vi "LaserPIDPositioning.vi"(0 "Servo Device In":i32, 1 "Vertical Edge":T1 {"Point2 (Real-World)"."Y" format="%.2f"; "Point2 (Real-World)"."X" format="%.2f"; "Point1 (Real-World)"."Y" format="%.2f"; "Point1 (Real-World)"."X" format="%.2f"; "Point2 (Pixels)"."Y" format="%.2f"; "Point2 (Pixels)"."X" format="%.2f"; "Point1 (Pixels)"."Y" format="%.2f"; "Point1 (Pixels)"."X" format="%.2f"}, 2 "Horizontal Edge":T1 {"Point2 (Real-World)"."Y" format="%.2f"; "Point2 (Real-World)"."X" format="%.2f"; "Point1 (Real-World)"."Y" format="%.2f"; "Point1 (Real-World)"."X" format="%.2f"; "Point2 (Pixels)"."Y" format="%.2f"; "Point2 (Pixels)"."X" format="%.2f"; "Point1 (Pixels)"."Y" format="%.2f"; "Point1 (Pixels)"."X" format="%.2f"}, 4 "servo error in":errorcluster, 5 "error in":errorcluster, 8 "Destination Point":cluster{"DestinationX":dbl, "DestinationY":dbl}, 9 "Servo Angles In":cluster{"Angle X":dbl, "Angle Y":dbl}) -> (11 "Servo Angles Out":cluster{"Angle X":dbl, "Angle Y":dbl}, 14 "Servo Device Out":i32, 18 "servo error out":errorcluster, 19 "error out":errorcluster)   [LabVIEW 2014]
uses:
  <vilib>/addons/control/pid/pid.llb/PID (DBL).vi
  <vilib>/vision/NI_Vision_Development_Module.lvlib
  <vilib>/addons/control/pid/NI_PID_pid.lvlib
panel:
  out "x+y 2":dbl
  out "x+y":dbl
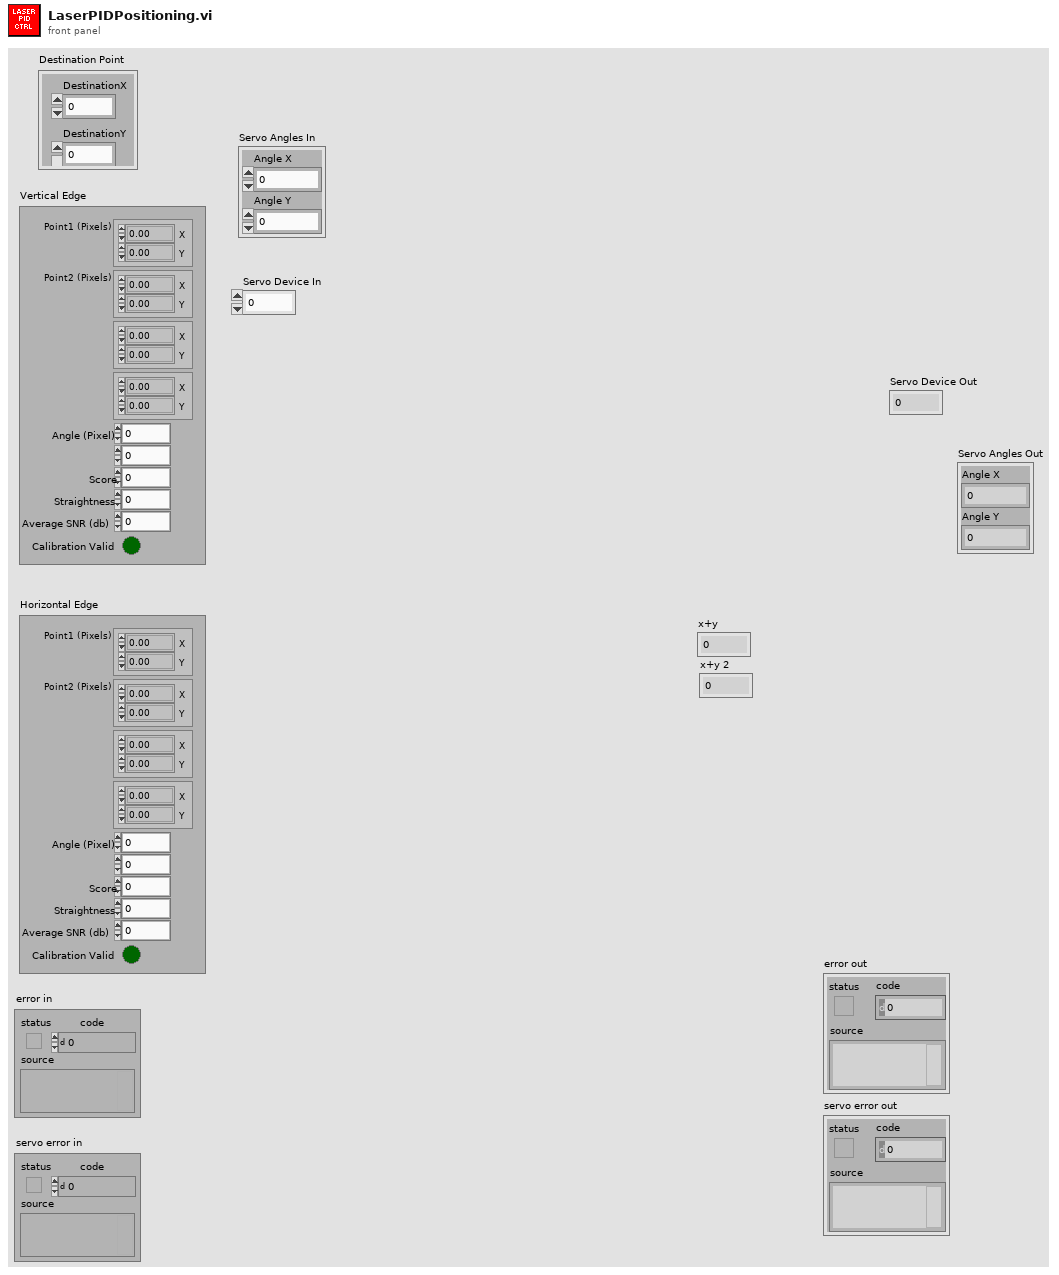
[diagram p1: front panel]
types:
  T1 = cluster{"Point1 (Pixels)":cluster{"X":sgl, "Y":sgl}, "Point2 (Pixels)":cluster{"X":sgl, "Y":sgl}, "Point1 (Real-World)":cluster{"X":sgl, "Y":sgl}, "Point2 (Real-World)":cluster{"X":sgl, "Y":sgl}, "Angle (Pixel)":dbl, "Angle (Real-World)":dbl, "Score":dbl, "Straightness":dbl, "Average SNR (db)":dbl, "Calibration Valid":bool}
  T2 = cluster{"proportional gain (Kc)":dbl, "integral time (Ti, min)":dbl, "derivative time (Td, min)":dbl}
  T3 = cluster{cluster{"X":sgl, "Y":sgl}, cluster{"X":sgl, "Y":sgl}}
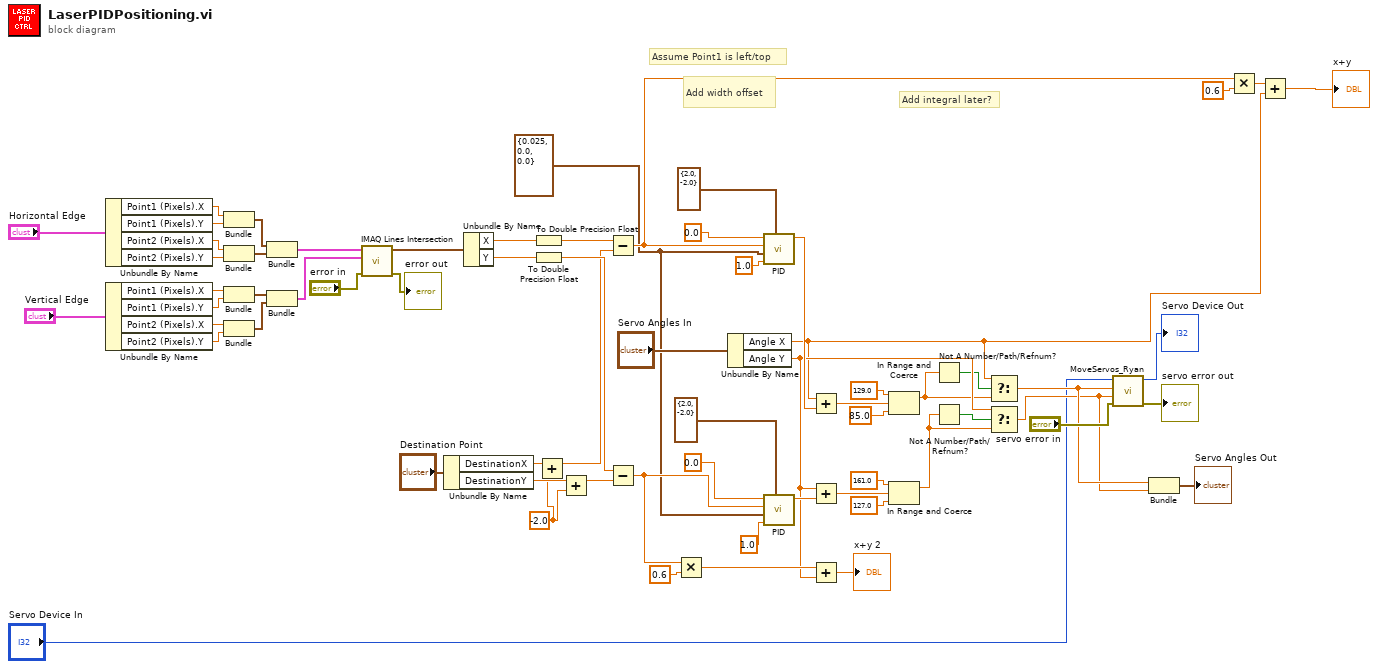
[diagram p0: block diagram]
diagram:
  w1 = -2.0 ("y")
  w4 = T2 {"proportional gain (Kc)"=0.025, "integral time (Ti, min)"=0.0, "derivative time (Td, min)"=0.0} ("PID gains")
  # "Add integral later?"
  # "Add width offset"
  # "Assume Point1 is left/top"
  n1 = Unbundle By Name("Horizontal Edge") -> ("Point1 (Pixels).X"=w63:sgl, "Point1 (Pixels).Y"=w62:sgl, "Point2 (Pixels).X"=w61:sgl, "Point2 (Pixels).Y"=w60:sgl)
  n2 = Unbundle By Name("Vertical Edge") -> ("Point1 (Pixels).X"=w54:sgl, "Point1 (Pixels).Y"=w53:sgl, "Point2 (Pixels).X"=w52:sgl, "Point2 (Pixels).Y"=w51:sgl)
  n3 = Bundle("X"=w63, "Y"=w62) -> (w59:cluster{"X":sgl, "Y":sgl})  [unwired: 1 in]
  n4 = Bundle("X"=w61, "Y"=w60) -> (w58:cluster{"X":sgl, "Y":sgl})  [unwired: 1 in]
  n5 = Bundle("X"=w54, "Y"=w53) -> (w56:cluster{"X":sgl, "Y":sgl})  [unwired: 1 in]
  n6 = Bundle("X"=w52, "Y"=w51) -> (w55:cluster{"X":sgl, "Y":sgl})  [unwired: 1 in]
  n7 = Bundle(w59, w58) -> (w57:T3)  [unwired: 1 in]
  n8 = Bundle(w56, w55) -> (w50:T3)  [unwired: 1 in]
  n9 = call "IMAQ Lines Intersection"("error in (no error)"="error in", "Line 2"=w50, "Line 1"=w57) -> ("error out"=→"error out":errorcluster, "Intersection Point"=w48:cluster{"X":sgl, "Y":sgl})  [unwired: 6 in, 1 out]
  n10 = Unbundle By Name("Destination Point") -> ("DestinationX"=w45:dbl, "DestinationY"=w41:dbl)
  n11 = Unbundle By Name(w48) -> ("X"=w38:sgl, "Y"=w42:sgl)
  n12 = To Double Precision Float(number=w38) -> (double precision float=w27:dbl)
  n13 = To Double Precision Float(number=w42) -> (double precision float=w37:dbl)
  n14 = Add(x=w45, y=w1) -> (x+y=w3:dbl)
  n15 = Add(x=w41, y=w1) -> (x+y=w2:dbl)
  n16 = Subtract(x=w27, y=w3) -> (x-y=w25:dbl)
  n17 = Subtract(x=w37, y=w2) -> (x-y=w22:dbl)
  n18 = Multiply(x=w22, y=0.6) -> (x*y=w21:dbl)
  n19 = Unbundle By Name("Servo Angles In") -> ("Angle X"=w10:dbl, "Angle Y"=w13:dbl)
  n20 = call-poly <vilib>:"PID.vi"("output range"=cluster{"output high":dbl, "output low":dbl} {"output high"=2.0, "output low"=-2.0}, "dt (s)"=1.0, "PID gains"=w4, "process variable"=w25, "setpoint"=0.0) -> ("output"=w16:dbl)  [unwired: 5 in, 1 out]
  n21 = call-poly <vilib>:"PID.vi"("output range"=cluster{"output high":dbl, "output low":dbl} {"output high"=2.0, "output low"=-2.0}, "dt (s)"=1.0, "PID gains"=w4, "process variable"=w22, "setpoint"=0.0) -> ("output"=w18:dbl)  [unwired: 5 in, 1 out]
  n22 = Add(x=w10, y=w16) -> (x+y=w15:dbl)
  n23 = Add(x=w13, y=w18) -> (x+y=w17:dbl)
  n24 = Add(x=w21, y=w13) -> (x+y=→"x+y 2":dbl)
  n25 = In Range and Coerce(upper limit=129.0, x=w15, lower limit=85.0) -> (coerced(x)=w9:dbl)  [unwired: 1 out]
  n26 = In Range and Coerce(upper limit=161.0, x=w17, lower limit=127.0) -> (coerced(x)=w12:dbl)  [unwired: 1 out]
  n27 = Not A Number/Path/Refnum?(number/path/refnum=w9) -> (NaN/Path/Refnum?=w11:bool)
  n28 = Not A Number/Path/Refnum?(number/path/refnum=w12) -> (NaN/Path/Refnum?=w14:bool)
  n29 = Select(t=w10, s=w11, f=w9) -> (s? t:f=w8:dbl)
  n30 = Select(t=w13, s=w14, f=w12) -> (s? t:f=w7:dbl)
  n31 = call "MoveServos_Ryan.vi"("servo error in"="servo error in", "Y pos"=w7, "X pos"=w8, "Device In"="Servo Device In") -> ("servo error out"=→"servo error out":errorcluster, "Device Out"=→"Servo Device Out":i32)  [unwired: 6 in]
  n32 = Bundle("upper limit"=w8, "upper limit"=w7) -> (→"Servo Angles Out":cluster{"upper limit":dbl, "upper limit":dbl})  [unwired: 1 in]
  n33 = Multiply(x=w25, y=0.6) -> (x*y=w24:dbl)
  n34 = Add(x=w24, y=w10) -> (x+y=→"x+y":dbl)
